vi "mobileye2ethernet.vi"() -> ()   [LabVIEW 2015]
uses:
  <vilib>/FPGAPlugInAG/cRIO-9030/niLvFpga_Open_cRIO-9030.vi
  <vilib>/rvi/interface/common/dynamic/niFpgaDynamicAddResources.vi
  <vilib>/FPGAPlugInAG/Dynamic/niLvFpga_Abort_Dynamic.vi
  <vilib>/FPGAPlugInAG/Dynamic/niLvFpga_Run_Dynamic.vi
  <vilib>/Utility/error.llb/Error Cluster From Error Code.vi
  <vilib>/rvi/errors/niLvFpgaAdjustHostInterfaceError.vi
  rio_Global.vi
  <vilib>/rvi/interface/nirviOpenFPGA/nirviOpenFPGA.xnode
  FPGA Bitfiles/autonomous_FPGATarget4_fpga1_rudp+OsNkSQ.lvbitx
  fpga 1.vi
  <vilib>/rvi/interface/nirviMethod/nirviMethod.xnode
  <vilib>/FPGAPlugInAG/Dynamic/niLvFpga_ReadFifo_Dynamic.vi
  <vilib>/rvi/errors/niLvFpgaMergeErrorWithErrorCode.vi
panel:
  out "FPGA":refnum<k20>
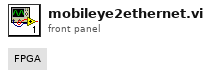
[diagram p1: front panel]
types:
  T1 = cluster{"connection ID":refnum<k16>, "net address":u32, "port":u16}
  T2 = cluster{"hash":i64, "sys time":i64, "mobileye time":u32, "ID":u32, "data":u8[]}
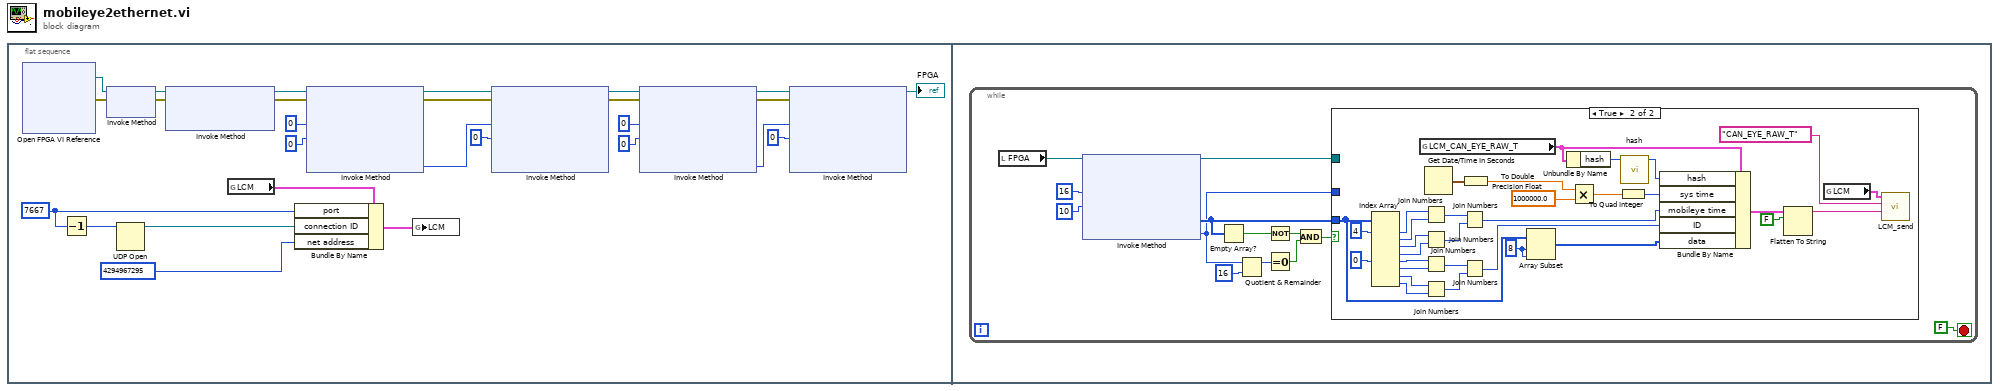
[diagram p0: block diagram]
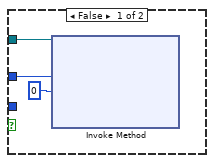
[diagram p2: hidden frame]
diagram:
  n1 = flat-sequence {
    frame #0 {
      w5 = u16 7667 ("port")
      n2 = xnode "Open FPGA VI Reference"() -> ("FPGA VI Reference Out"=w27:refnum<k20>, "error out"=w26:errorcluster)  [unwired: 2 in]
      n3 = Decrement(x=w5) -> (x-1=w6:u16)
      n4 = xnode "Invoke Method"("FPGA VI Reference In"=w27, "error in"=w26) -> ("FPGA VI Reference Out"=w25:refnum<k20>, "error out"=w24:errorcluster)
      n5 = UDP Open(11:w6) -> (port=w3:refnum<k16>)  [unwired: 4 in, 2 out]
      n6 = xnode "Invoke Method"("FPGA VI Reference In"=w25, "error in"=w24) -> ("FPGA VI Reference Out"=w23:refnum<k20>, "error out"=w22:errorcluster)  [unwired: 1 in]
      n7 = global read "rio_Global.vi" "LCM"() -> (w1:T1)
      n8 = Bundle By Name(cluster=w1, "port"=w5, "connection ID"=w3, "net address"=u32 4294967295) -> (w2:T1)
      n9 = xnode "Invoke Method"("FPGA VI Reference In"=w23, "error in"=w22, "Number of Elements"=u32 0, "Timeout (ms)"=0) -> ("FPGA VI Reference Out"=w19:refnum<k20>, "error out"=w18:errorcluster, "Elements Remaining"=w20:u32)  [unwired: 1 out]
      n10 = global write "rio_Global.vi" "LCM"(w2) -> ()
      n11 = xnode "Invoke Method"("FPGA VI Reference In"=w19, "error in"=w18, "Number of Elements"=w20, "Timeout (ms)"=0) -> ("FPGA VI Reference Out"=w9:refnum<k20>, "error out"=w8:errorcluster)  [unwired: 2 out]
      n12 = xnode "Invoke Method"("FPGA VI Reference In"=w9, "error in"=w8, "Number of Elements"=u32 0, "Timeout (ms)"=0) -> ("FPGA VI Reference Out"=w12:refnum<k20>, "error out"=w13:errorcluster, "Elements Remaining"=w11:u32)  [unwired: 1 out]
      n13 = xnode "Invoke Method"("FPGA VI Reference In"=w12, "error in"=w13, "Number of Elements"=w11, "Timeout (ms)"=0) -> ("FPGA VI Reference Out"=→"FPGA":refnum<k20>)  [unwired: 3 out]
    }
    frame #1 {
      n14 = while {
        stop <- FALSE stop-if-true
        n15 = local read "FPGA"() -> (w39:refnum<k20>)
        n16 = xnode "Invoke Method"("FPGA VI Reference In"=w39, "Number of Elements"=u32 16, "Timeout (ms)"=10) -> ("FPGA VI Reference Out"=w29:refnum<k20>, "Data"=w36:u8[], "Elements Remaining"=w28:u32)  [unwired: 1 in, 1 out]
        n17 = Empty Array?(array=w36) -> (empty?=w33:bool)
        n18 = Quotient & Remainder(x=w28, y=u32 16) -> (x-y*floor(x/y)=w34:u32)  [unwired: 1 out]
        n19 = Not(x=w33) -> (.not. x?=w32:bool)
        n20 = Equal To 0?(x=w34) -> (x = 0?=w31:bool)
        n21 = And(x=w32, y=w31) -> (x .and. y?=w30:bool)
        n22 = case shown="True" w30 {
          tunnel: w36 -> [_ w75]
          tunnel: w29 -> [w43 _]
          tunnel: w28 -> [w42 _]
          frame False {
            n23 = xnode "Invoke Method"("FPGA VI Reference In"=w43, "Number of Elements"=w42, "Timeout (ms)"=0) -> ()  [unwired: 1 in, 4 out]
          }
          frame True {
            w44 = 8 ("index")
            n24 = Index Array(array=w75, index #1=4 ("index"), index #5=0 ("index")) -> (element #1=w65:u8, element #2=w64:u8, element #3=w63:u8, element #4=w62:u8, element #5=w55:u8, element #6=w56:u8, element #7=w54:u8, element #8=w53:u8)  [unwired: 6 in]
            n25 = global read "rio_Global.vi" "LCM_CAN_EYE_RAW_T"() -> (w73:T2)
            n26 = Join Numbers(hi=w65, lo=w64) -> ((hi.lo)=w61:u16)
            n27 = Join Numbers(hi=w63, lo=w62) -> ((hi.lo)=w60:u16)
            n28 = Join Numbers(hi=w55, lo=w56) -> ((hi.lo)=w57:u16)
            n29 = Join Numbers(hi=w54, lo=w53) -> ((hi.lo)=w58:u16)
            n30 = Get Date/Time In Seconds() -> (seconds since 1Jan1904=w71:timestamp)
            n31 = Join Numbers(hi=w61, lo=w60) -> ((hi.lo)=w45:u32)
            n32 = Join Numbers(hi=w57, lo=w58) -> ((hi.lo)=w52:u32)
            n33 = To Double Precision Float(number=w71) -> (double precision float=w68:dbl)
            n34 = Array Subset(array=w75, index=w44, length=w44) -> (w51:u8[])
            n35 = Unbundle By Name(w73) -> ("hash"=w74:i64)
            n36 = Multiply(x=w68, y=1000000.0) -> (x*y=w69:dbl)
            n37 = To Quad Integer(1:w69) -> (0:w67:i64)
            n38 = call "hash.vi"("input"=w74) -> ("output"=w72:i64)  [unwired: 10 in]
            n39 = Bundle By Name(cluster=w73, "hash"=w72, "sys time"=w67, "mobileye time"=w45, "ID"=w52, "data"=w51) -> (w49:T2)
            n40 = Flatten To String(anything=w49, prepend array or string size? (T)=FALSE) -> (data string=w47:string)  [unwired: 2 in, 2 out]
            n41 = global read "rio_Global.vi" "LCM"() -> (w48:T1)
            n42 = call "LCM_send.vi"("DATA"=w47, "ID"="CAN_EYE_RAW_T", "LCM"=w48) -> ()  [unwired: 6 in, 3 out]
          }
        }
      }
    }
  }
